vi "tearDown.vi"() -> ()   [LabVIEW 2013, in "No Object Control TestCase.lvclass"]
uses:
  No Object Control TestCase.lvclass
panel:
  out "No Object Control TestCase.lvclass 2":refnum<class "No Object Control TestCase.lvclass">
  in  "No Object Control TestCase.lvclass":refnum<class "No Object Control TestCase.lvclass">
  out "error out":errorcluster
  in  "error in (no error)":errorcluster
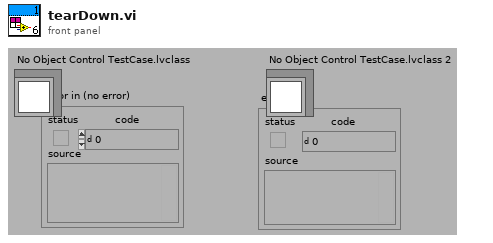
[diagram p1: front panel]
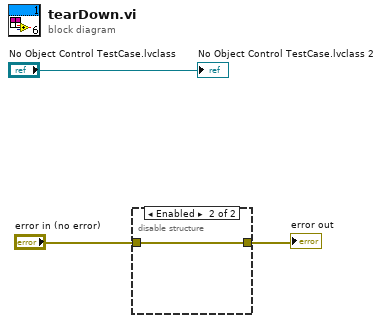
[diagram p0: block diagram]
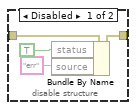
[diagram p2: hidden frame]
diagram:
  n1 = disable-structure shown="Enabled" {
    disable-tunnel: "error in (no error)" -> [w7 w8]
    disable-tunnel: [w6 w8] -> w2
    frame Disabled {
      n2 = Bundle By Name(cluster=w7, "status"=TRUE, "source"="err") -> (w6:errorcluster)
    }
    frame Enabled {
    }
  }
  "error out" <- w2
  "No Object Control TestCase.lvclass 2" <- "No Object Control TestCase.lvclass"
